vi "Robotics Environment Simulator.vi"() -> ()   [LabVIEW 2012]
doc: "This VI starts and stops the environment simulator and serves as the master VI for your simulation code. Open and run this VI to display the environment simulator, or open the block diagram to view or modify simulation code."
uses:
  <vilib>/robotics/Simulator/NI_Robotics_Simulator.lvlib
panel:
  in  "manifest filename":string="Robotics Environment Simulator.xml"
  in  "stop":bool
  # "* Press the Run button to display the Robotics Environment Simulator.\n* Select Window>>Show Block Diagram or press <Ctrl-E> to view the block diagram, where you can add or modify simulation code. Add controls and indicators to the front panel of this VI to pass data into and out of the simulation code.\n* The manifest file must exist in same directory as the .lvproj file."
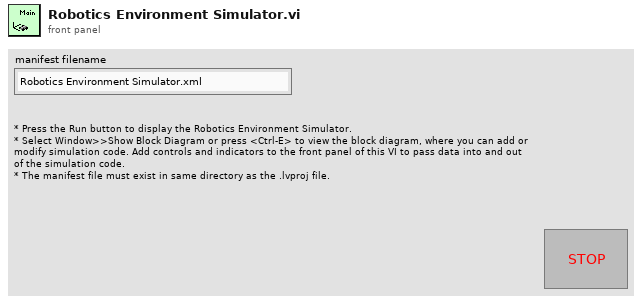
[diagram p1: front panel]
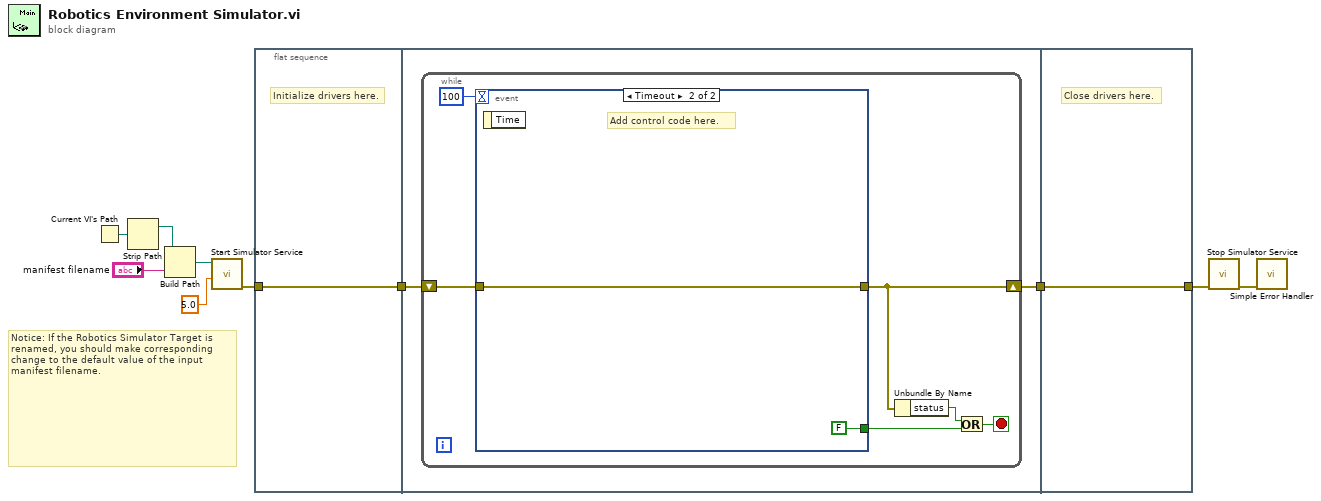
[diagram p0: block diagram]
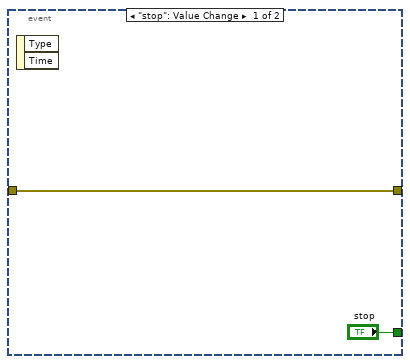
[diagram p2: hidden frame]
diagram:
  # "Notice: If the Robotics Simulator Target is renamed, you should make corresponding change to the default value of the input manifest filename."
  n1 = Current VI's Path() -> (path=w8:path)
  n2 = Strip Path(path=w8) -> (stripped path=w7:path)  [unwired: 1 out]
  n3 = Build Path(base path=w7, name or relative path="manifest filename") -> (appended path=w6:path)
  n4 = call <vilib>:"Start Simulator Service.vi"("step size (ms)"=5.0 ("stepsize(ms)"), "manifest file"=w6) -> ("error out"=w3:errorcluster)  [unwired: 9 in]
  n5 = flat-sequence {
    tunnel: w3 -> [w11]
    tunnel: [w11] -> w2
    tunnel: w2 -> [w12]
    tunnel: [w13] -> w1
    tunnel: [w24] -> w9
    tunnel: w1 -> [w24]
    frame #0 {
      # "Initialize drivers here."
    }
    frame #1 {
      n6 = while {
        shift-right: [w15] -> w13
        shift-left: w12 -> [w18]
        stop <- w16 stop-if-true
        n7 = event shown="[1] Timeout" {
          selector: _ -> [_ _]
          dyn-events: _ -> [_ _]
          timeout: 100 -> [_ _]
          tunnel: ["stop" FALSE ("stop")] -> w17
          tunnel: [w20 w23] -> w15
          tunnel: w18 -> [w20 w23]
          event "stop": Value Change {
            n8 = event-data() -> ()  [unwired: 1 in, 2 out]
          }
          event Timeout {
            # "Add control code here."
            n9 = event-data() -> ()  [unwired: 1 in, 1 out]
          }
        }
        n10 = Unbundle By Name(w15) -> ("status"=w14:bool)
        n11 = Or(x=w14, y=w17) -> (x .or. y?=w16:bool)
      }
    }
    frame #2 {
      # "Close drivers here."
    }
  }
  n12 = call <vilib>:"Stop Simulator Service.vi"("error in (no error)"=w9) -> ("error out"=w4:errorcluster)  [unwired: 10 in]
  n13 = call <vilib>:"Simple Error Handler.vi"("error in (no error)"=w4) -> ()  [unwired: 4 in, 5 out]
